vi "JAVA_DriveState.vi"   [LabVIEW 2016]
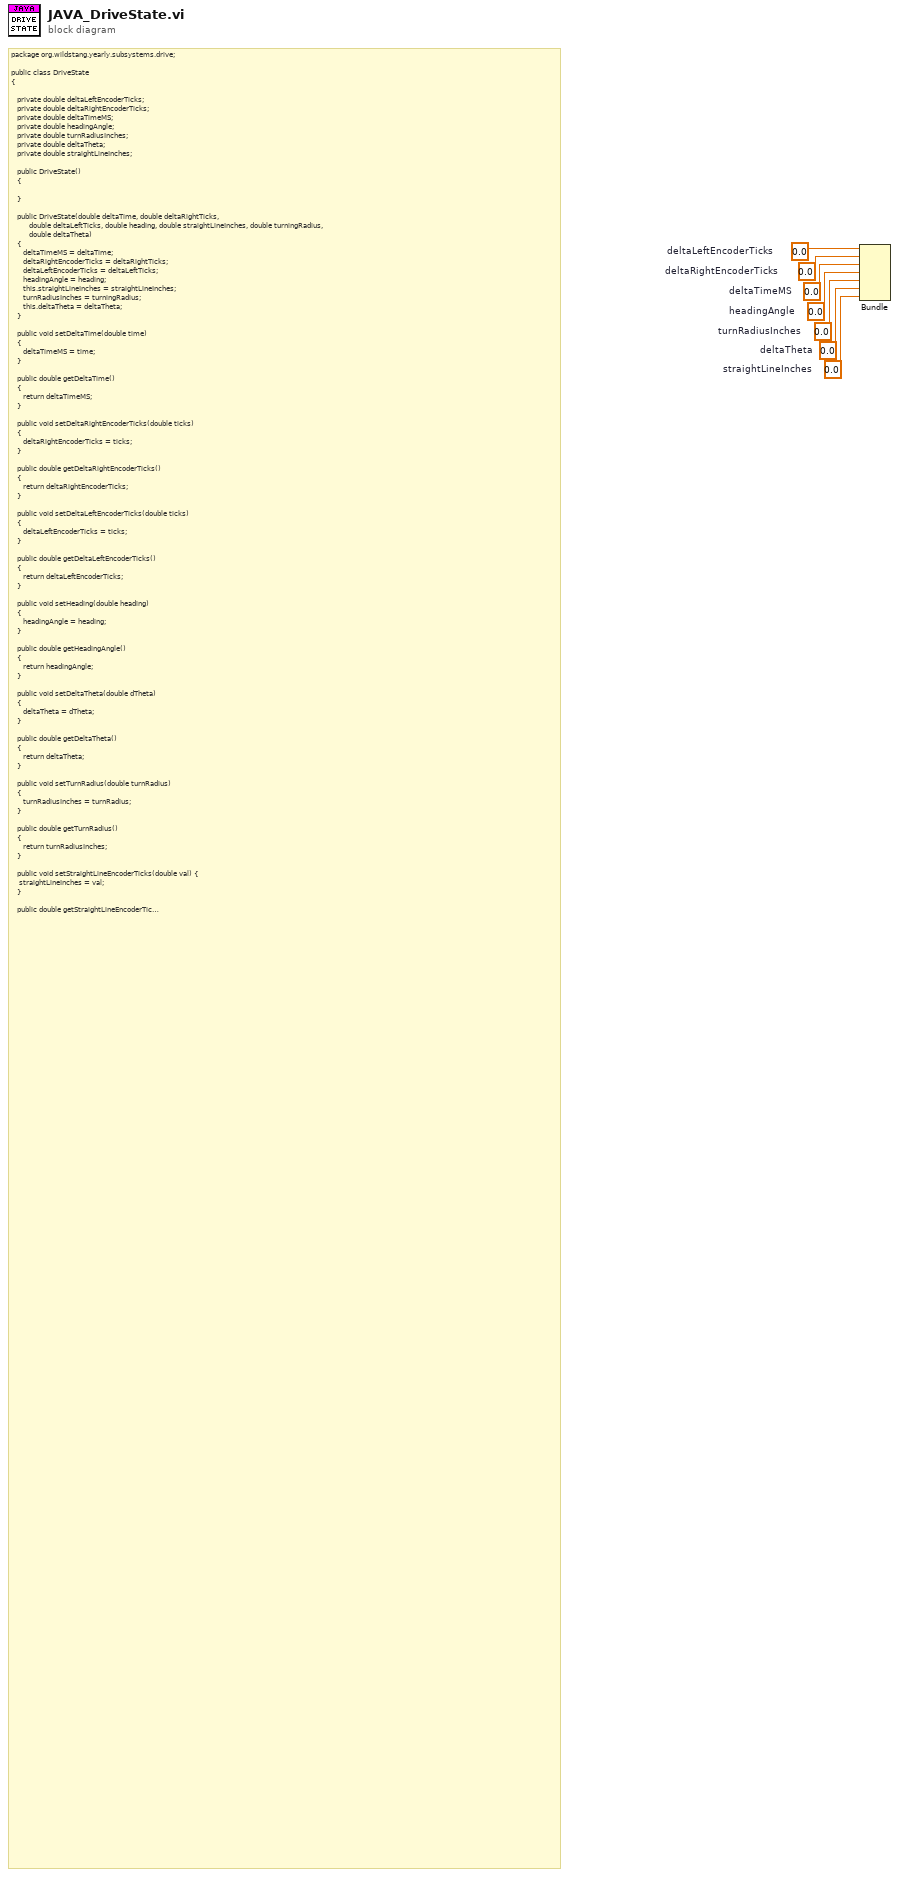
[diagram p0: block diagram]
diagram:
  w1 = 0.0  # straightLineInches
  w2 = 0.0  # deltaTheta
  w3 = 0.0  # turnRadiusInches
  w4 = 0.0  # headingAngle
  w5 = 0.0  # deltaTimeMS
  w6 = 0.0  # deltaRightEncoderTicks
  w7 = 0.0  # deltaLeftEncoderTicks
  # "package org.wildstang.yearly.subsystems.drive;\n\npublic class DriveState\n{\n\n   private double deltaLeftEncoderTicks;\n   private double deltaRightEncoderTicks;\n   private double deltaTimeMS;\n   private double headingAngle;\n   private double turnRadiusInches;\n   private double deltaTheta;\n   private double straightLineInches;\n\n   public DriveState()\n   {\n\t   \n   }\n\n   public DriveState(double deltaTime, double deltaRightTicks,\n         double deltaLeftTicks, double heading, double straightLineInches, double turningRadius,\n         double deltaTheta)\n   {\n      deltaTimeMS = deltaTime;\n      deltaRightEncoderTicks = deltaRightTicks;\n      deltaLeftEncoderTicks = deltaLeftTicks;\n      headingAngle = heading;\n      this.straightLineInches = straightLineInches;\n      turnRadiusInches = turningRadius;\n      this.deltaTheta = deltaTheta;\n   }\n\n   public void setDeltaTime(double time)\n   {\n      deltaTimeMS = time;\n   }\n\n   public double getDeltaTime()\n   {\n      return deltaTimeMS;\n   }\n\n   public void setDeltaRightEncoderTicks(double ticks)\n   {\n      deltaRightEncoderTicks = ticks;\n   }\n\n   public double getDeltaRightEncoderTicks()\n   {\n      return deltaRightEncoderTicks;\n   }\n\n   public void setDeltaLeftEncoderTicks(double ticks)\n   {\n      deltaLeftEncoderTicks = ticks;\n   }\n\n   public double getDeltaLeftEncoderTicks()\n   {\n      return deltaLeftEncoderTicks;\n   }\n\n   public void setHeading(double heading)\n   {\n      headingAngle = heading;\n   }\n\n   public double getHeadingAngle()\n   {\n      return headingAngle;\n   }\n\n   public void setDeltaTheta(double dTheta)\n   {\n      deltaTheta = dTheta;\n   }\n\n   public double getDeltaTheta()\n   {\n      return deltaTheta;\n   }\n\n   public void setTurnRadius(double turnRadius)\n   {\n      turnRadiusInches = turnRadius;\n   }\n\n   public double getTurnRadius()\n   {\n      return turnRadiusInches;\n   }\n\n   public void setStraightLineEncoderTicks(double val) {\n\t   straightLineInches = val;\n   }\n   \n   public double getStraightLineEncoderTicks() {\n\t   return straightLineInches;\n   }\n   \n   public String toString()\n   {\n      return deltaTimeMS + \", \" + deltaRightEncoderTicks + \", \"\n            + deltaLeftEncoderTicks + \", \" + headingAngle + \", \" + \n            straightLineInches + \", \" + turnRadiusInches + \", \" + deltaTheta + \"\\n\";\n   }\n\n}"
  n1 = Bundle("deltaLeftEncoderTicks"=w7, "deltaRightEncoderTicks"=w6, "deltaTimeMS"=w5, "headingAngle"=w4, "turnRadiusInches"=w3, "deltaTheta"=w2, "straightLineInches"=w1) -> ()  [unwired: 1 in, 1 out]
